vi "Version_4.9_8_on-chip_valves_for25ulSyringe_withModfied_Plunging.vi"() -> ()   [LabVIEW 2020] (continued)
                                n336 = local read "VISA Refnum in\nfor Pump"() -> (w823:refnum<visa-resource-name>)
                                n337 = call "HardStopCurrentProcess (SubVI).vi"("VISA Refnum in"=w823) -> ()  [unwired: 11 in]
                                }
                              }
                              n338 = local read "VISA Refnum in\nfor Pump"() -> (w821:refnum<visa-resource-name>)
                              n339 = call "ProcessCompletionWaiter (SubVI).vi"("VISA Refnum in"=w821) -> ()  [unwired: 11 in]
                            }
                          }
                        }
                      }
                      frame #1 {
                        n340 = local write "Start the Process"(FALSE ("Start the Process")) -> ()
                      }
                    }
                  }
                }
              }
              frame True {
                n341 = local write "Pause Data Collection"(FALSE ("Pause Data Collection")) -> ()
              }
            }
          }
          frame "Initialize Only The Pump" {
            n342 = local read "Stop for End of \nExperiment \nand Data Writing"() -> (w826:bool)
            n343 = case shown="False" w826 {
              frame False {
                n344 = local read "Start the Process"() -> (w827:bool)
                n345 = case shown="True" w827 {
                  frame False {
                    n346 = local read "Stopper that ends \nthe main loops"() -> (w829:bool)
                    n347 = local read "Start the Process"() -> (w830:bool)
                    n348 = Or(x=w830, y=w829) -> (x .or. y?=w828:bool)
                    n349 = case shown="False" w828 {
                      frame False {
                        n350 = while {
                          stop <- w833 stop-if-true
                          n351 = local read "Stopper that ends \nthe main loops"() -> (w835:bool)
                          n352 = local read "Start the Process"() -> (w834:bool)
                          n353 = Or(x=w834, y=w835) -> (x .or. y?=w833:bool)
                          n354 = Wait (ms)(milliseconds to wait=u32 10) -> ()  [unwired: 1 out]
                        }
                        n355 = One Button Dialog(message="Please select the process and press the 'Start Process' Button") -> ()  [unwired: 1 in, 1 out]
                      }
                      frame True {
                      }
                    }
                  }
                  frame True {
                    n356 = stacked-sequence {
                      frame #0 {
                        n357 = local read "VISA Refnum in\nfor Pump"() -> (w836:refnum<visa-resource-name>)
                        n358 = call "Initializer (SubVI).vi"("VISA Refnum in"=w836) -> ()  [unwired: 11 in]
                      }
                      frame #1 {
                        n359 = local read "VISA Refnum in\nfor Pump"() -> (w837:refnum<visa-resource-name>)
                        n360 = call "ProcessCompletionWaiter (SubVI).vi"("VISA Refnum in"=w837) -> ()  [unwired: 11 in]
                      }
                      frame #2 {
                        n361 = local write "Start the Process"(FALSE ("Start the Process")) -> ()
                      }
                    }
                  }
                }
              }
              frame True {
              }
            }
          }
          frame "Automated Protein Purification with 7 SOD Valves and On/Off External Valve" {
            n362 = local read "Stopper that ends \nthe main loops"() -> (w839:bool)
            n363 = case shown="False" w839 {
              frame False {
                n364 = local read "Start the Process"() -> (w840:bool)
                n365 = case shown="True" w840 {
                  frame False {
                    n366 = local read "Stopper that ends \nthe main loops"() -> (w842:bool)
                    n367 = local read "Start the Process"() -> (w841:bool)
                    n368 = Or(x=w842, y=w841) -> (x .or. y?=w843:bool)
                    n369 = case shown="False" w843 {
                      frame False {
                        n370 = while {
                          stop <- w846 stop-if-true
                          n371 = local read "Stop for End of \nExperiment \nand Data Writing"() -> (w845:bool)
                          n372 = local read "Stopper that ends \nthe main loops"() -> (w848:bool)
                          n373 = local read "Start the Process"() -> (w847:bool)
                          n374 = Wait (ms)(milliseconds to wait=u32 10) -> ()  [unwired: 1 out]
                          n375 = Or(x=w848, y=w847) -> (x .or. y?=w846:bool)
                          n376 = local write "Stopper that ends \nthe main loops"(w845) -> ()
                        }
                        n377 = One Button Dialog(message="Please Select the Process and Press 'Start the Process' Button") -> ()  [unwired: 1 in, 1 out]
                      }
                      frame True {
                      }
                    }
                  }
                  frame True {
                    n378 = stacked-sequence {
                      frame #0 {
                        # "Equilibrate Column-1 with Buffer-A obtained from port-4 and pumped via port-2 and Column-2 with Buffer-C obtained from port-4 and pumped onto chip via port-6 onto the chip ...with an initial and inbetween wash of tubings while changing the buffers"
                        n379 = stacked-sequence {
                          frame #0 {
                            n380 = local read "VISA Refnum in\nfor Valve"() -> (w857:refnum<visa-resource-name>)
                            n381 = local read "External Valve \nCLOSED"() -> (w856:string)
                            n382 = local write "Valve V4 Open"(FALSE ("Valve V4 Open")) -> ()
                            n383 = local write "Valve V1 Open"(FALSE ("Valve V1 Open")) -> ()
                            n384 = local write "Valve V2 Open"(FALSE ("Valve V2 Open")) -> ()
                            n385 = local write "Valve V3 Open"(FALSE ("Valve V3 Open")) -> ()
                            n386 = call "PortChanger_Valve (SubVI).vi"("Port Number"=w856, "VISA Refnum in"=w857) -> ()  [unwired: 10 in]
                            n387 = local write "Valve V7 Open"(FALSE ("Valve V7 Open")) -> ()
                            n388 = local write "Valve V5 Open"(FALSE ("Valve V5 Open")) -> ()
                            n389 = local write "Valve V6 Open"(FALSE ("Valve V6 Open")) -> ()
                            n390 = call <vilib>:"fgt init.vi"() -> ("error out"=w852:errorcluster)  [unwired: 11 in]
                            n391 = while {
                              tunnel: w852 -> [w863]
                              tunnel: [w862] -> w851
                              stop <- w866 stop-if-true
                              # "Keeping the valve closing pressure of push pull to zero"
                              n392 = local read "Stop for End of \nExperiment \nand Data Writing"() -> (w867:bool)
                              n393 = local read "Equilibriating \nColumn-1"() -> (w868:bool)
                              n394 = call <vilib>:"fgt set pressure.vi"("error in (no error)"=w863, "pressure"=sgl 0.0 ("order"), "pressureIndex"=1 ("module")) -> ("error out"=w862:errorcluster)  [unwired: 8 in]
                              n395 = Or(x=w868, y=w867) -> (x .or. y?=w866:bool)
                              n396 = Wait (ms)(milliseconds to wait=u32 10) -> ()  [unwired: 1 out]
                            }
                            n397 = call <vilib>:"fgt close.vi"("error in (no error)"=w851) -> ()  [unwired: 10 in, 1 out]
                          }
                          frame #1 {
                            # "Clean the tubing with Buffer-A1"
                            n398 = local read "N-A1"() -> (w870:i32)
                            n399 = for {
                              N: w870 -> [_]
                              n400 = stacked-sequence {
                                frame #0 {
                                n401 = local read "VISA Refnum in\nfor Pump"() -> (w873:refnum<visa-resource-name>)
                                n402 = local read "Port for \nA1-Equilibriation"() -> (w872:string)
                                n403 = call "PortChanger (SubVI).vi"("Port Number"=w872, "VISA Refnum in"=w873) -> ()  [unwired: 10 in]
                                }
                                frame #1 {
                                n404 = local read "VISA Refnum in\nfor Pump"() -> (w874:refnum<visa-resource-name>)
                                n405 = call "ProcessCompletionWaiter (SubVI).vi"("VISA Refnum in"=w874) -> ()  [unwired: 11 in]
                                }
                                frame #2 {
                                n406 = local read "VISA Refnum in\nfor Pump"() -> (w879:refnum<visa-resource-name>)
                                n407 = local read "Apparent Volume\nof Syringe"() -> (w875:dbl)
                                n408 = local read "Volume of Syringe"() -> (w876:dbl)
                                n409 = call "RPickUp(SubVI).vi"("Volume to be picked up"=w875, "Volume of Syringe"=w876, "Resolution of PickUP"=T2."Standard Pumping", "PickUp Flow Rate (ul/min)"=150.0, "VISA Refnum in"=w879) -> ()  [unwired: 6 in, 1 out]
                                }
                                frame #3 {
                                n410 = local read "Stopper that ends \nthe main loops"() -> (w880:bool)
                                n411 = local read "VISA Refnum in\nfor Pump"() -> (w881:refnum<visa-resource-name>)
                                n412 = case shown="True" w880 {
                                frame False {
                                }
                                frame True {
                                n413 = local read "VISA Refnum in\nfor Pump"() -> (w882:refnum<visa-resource-name>)
                                n414 = call "HardStopCurrentProcess (SubVI).vi"("VISA Refnum in"=w882) -> ()  [unwired: 11 in]
                                }
                                }
                                n415 = call "ProcessCompletionWaiter (SubVI).vi"("VISA Refnum in"=w881) -> ()  [unwired: 11 in]
                                }
                                frame #4 {
                                n416 = local read "VISA Refnum in\nfor Pump"() -> (w884:refnum<visa-resource-name>)
                                n417 = call "PortChanger (SubVI).vi"("Port Number"="1", "VISA Refnum in"=w884) -> ()  [unwired: 10 in]
                                }
                                frame #5 {
                                n418 = local read "Stopper that ends \nthe main loops"() -> (w885:bool)
                                n419 = local read "VISA Refnum in\nfor Pump"() -> (w886:refnum<visa-resource-name>)
                                n420 = case shown="True" w885 {
                                frame False {
                                }
                                frame True {
                                n421 = local read "VISA Refnum in\nfor Pump"() -> (w887:refnum<visa-resource-name>)
                                n422 = call "HardStopCurrentProcess (SubVI).vi"("VISA Refnum in"=w887) -> ()  [unwired: 11 in]
                                }
                                }
                                n423 = call "ProcessCompletionWaiter (SubVI).vi"("VISA Refnum in"=w886) -> ()  [unwired: 11 in]
                                }
                                frame #6 {
                                n424 = local read "VISA Refnum in\nfor Pump"() -> (w892:refnum<visa-resource-name>)
                                n425 = local read "Volume of Syringe"() -> (w889:dbl)
                                n426 = call "GoToAbsolutePosition(SubVI).vi"("Absolute Volume Position in Syringe (in ul)"=0.0 ("Volume to be picked up"), "Volume of Syringe"=w889, "Resolution of Pumping"=T2."Standard Pumping" ("Resolution of PickUP"), "Flow Rate (ul/min)"=150.0 ("PickUp Flow Rate (ul/min)"), "VISA Refnum in"=w892) -> ()  [unwired: 6 in, 1 out]
                                }
                                frame #7 {
                                n427 = local read "Stopper that ends \nthe main loops"() -> (w893:bool)
                                n428 = local read "VISA Refnum in\nfor Pump"() -> (w894:refnum<visa-resource-name>)
                                n429 = case shown="True" w893 {
                                frame False {
                                }
                                frame True {
                                n430 = local read "VISA Refnum in\nfor Pump"() -> (w895:refnum<visa-resource-name>)
                                n431 = call "HardStopCurrentProcess (SubVI).vi"("VISA Refnum in"=w895) -> ()  [unwired: 11 in]
                                }
                                }
                                n432 = call "ProcessCompletionWaiter (SubVI).vi"("VISA Refnum in"=w894) -> ()  [unwired: 11 in]
                                }
                              }
                              n433 = local write "Pause Data Collection"(TRUE ("Pause Data Collection")) -> ()
                            }
                          }
                          frame #2 {
                            # "Switch to Port-4"
                            # "Port-4 of pump is connected to Buffer-A1"
                            n434 = local read "Port for \nA1-Equilibriation"() -> (w896:string)
                            n435 = local read "VISA Refnum in\nfor Pump"() -> (w897:refnum<visa-resource-name>)
                            n436 = call "PortChanger (SubVI).vi"("Port Number"=w896, "VISA Refnum in"=w897) -> ()  [unwired: 10 in]
                          }
                          frame #3 {
                            n437 = local read "VISA Refnum in\nfor Pump"() -> (w898:refnum<visa-resource-name>)
                            n438 = call "ProcessCompletionWaiter (SubVI).vi"("VISA Refnum in"=w898) -> ()  [unwired: 11 in]
                          }
                          frame #4 {
                            n439 = local read "VISA Refnum in\nfor Valve"() -> (w905:refnum<visa-resource-name>)
                            n440 = local read "External Valve \nOPEN"() -> (w904:string)
                            n441 = local write "Valve V3 Open"(FALSE ("Valve V3 Open")) -> ()
                            n442 = local write "Valve V4 Open"(FALSE ("Valve V4 Open")) -> ()
                            n443 = local write "Valve V1 Open"(TRUE ("Valve V1 Open")) -> ()
                            n444 = local write "Valve V2 Open"(TRUE ("Valve V2 Open")) -> ()
                            n445 = call "PortChanger_Valve (SubVI).vi"("Port Number"=w904, "VISA Refnum in"=w905) -> ()  [unwired: 10 in]
                            n446 = local write "Valve V6 Open"(FALSE ("Valve V6 Open")) -> ()
                            n447 = local write "Valve V5 Open"(FALSE ("Valve V5 Open")) -> ()
                            n448 = local write "Valve V7 Open"(FALSE ("Valve V7 Open")) -> ()
                          }
                          frame #5 {
                            n449 = local read "Buffer-A1 Volume \nto be  Pumped \nfor Equilibration\nof Column-1"() -> (w911:dbl)
                            n450 = local read "Apparent Volume\nof Syringe"() -> (w908:dbl)
                            n451 = Quotient & Remainder(x=w911, y=w908) -> (x-y*floor(x/y)=w909:dbl, floor(x/y)=w910:dbl)
                            n452 = for {
                              N: w910 -> [_]
                              n453 = stacked-sequence {
                                frame #0 {
                                n454 = local read "Buffer-A1 PickUp \nFlow Rate (ul/min)\nfor Equilibration \nof Column-1"() -> (w914:dbl)
                                n455 = local read "Buffer-A1 Pumping\nResolution \nfor Equilibration \nof Column-1"() -> (w913:T2)
                                n456 = local read "VISA Refnum in\nfor Pump"() -> (w916:refnum<visa-resource-name>)
                                n457 = local read "Apparent Volume\nof Syringe"() -> (w912:dbl)
                                n458 = local read "Volume of Syringe"() -> (w915:dbl)
                                n459 = call "RPickUp(SubVI).vi"("Volume to be picked up"=w912, "Volume of Syringe"=w915, "Resolution of PickUP"=w913, "PickUp Flow Rate (ul/min)"=w914, "VISA Refnum in"=w916) -> ()  [unwired: 6 in, 1 out]
                                }
                                frame #1 {
                                n460 = while {
                                stop <- w917 stop-if-true
                                n461 = local read "Stopper that ends \nthe main loops"() -> (w918:bool)
                                n462 = local read "VISA Refnum in\nfor Pump"() -> (w919:refnum<visa-resource-name>)
                                n463 = case shown="True" w918 {
                                frame False {
                                }
                                frame True {
                                n464 = local read "VISA Refnum in\nfor Pump"() -> (w920:refnum<visa-resource-name>)
                                n465 = call "HardStopCurrentProcess (SubVI).vi"("VISA Refnum in"=w920) -> ()  [unwired: 11 in]
                                }
                                }
                                n466 = call "ProcessCompletionWaiterWithOutPut (SubVI).vi"("VISA Refnum in"=w919) -> ("Boolean"=w917:bool)  [unwired: 10 in]
                                }
                                }
                                frame #2 {
                                # "Reads the initial Plunger Position for computing the volume dispensed"
                                n467 = local read "VISA Refnum in\nfor Pump"() -> (w922:refnum<visa-resource-name>)
                                n468 = call "AbsolutePlungerPosition (SubVI).vi"("VISA Refnum in"=w922) -> ("Plunger Position"=w921:i32)  [unwired: 10 in]
                                n469 = local write "Initial Plunger Position"(w921) -> ()
                                }
                                frame #3 {
                                # "Switch to Port-2"
                                # "Port-2 of the pump is conncted to column-1 of chip"
                                n470 = local read "VISA Refnum in\nfor Pump"() -> (w924:refnum<visa-resource-name>)
                                n471 = call "PortChanger (SubVI).vi"("Port Number"="2", "VISA Refnum in"=w924) -> ()  [unwired: 10 in]
                                }
                                frame #4 {
                                n472 = while {
                                stop <- w925 stop-if-true
                                n473 = local read "Stopper that ends \nthe main loops"() -> (w926:bool)
                                n474 = local read "VISA Refnum in\nfor Pump"() -> (w927:refnum<visa-resource-name>)
                                n475 = case shown="True" w926 {
                                frame False {
                                }
                                frame True {
                                n476 = local read "VISA Refnum in\nfor Pump"() -> (w928:refnum<visa-resource-name>)
                                n477 = call "HardStopCurrentProcess (SubVI).vi"("VISA Refnum in"=w928) -> ()  [unwired: 11 in]
                                }
                                }
                                n478 = call "ProcessCompletionWaiterWithOutPut (SubVI).vi"("VISA Refnum in"=w927) -> ("Boolean"=w925:bool)  [unwired: 10 in]
                                }
                                }
                                frame #5 {
                                n479 = local read "Buffer-A1 Dispense\nFlow Rate (ul/min) \nfor Equilibration\nof Column-1"() -> (w932:dbl)
                                n480 = local read "Buffer-A1 Pumping\nResolution \nfor Equilibration \nof Column-1"() -> (w931:T2)
                                n481 = local read "VISA Refnum in\nfor Pump"() -> (w934:refnum<visa-resource-name>)
                                n482 = local write "Pause Data Collection"(FALSE ("Pause Data Collection")) -> ()
                                n483 = local read "Volume of Syringe"() -> (w933:dbl)
                                n484 = call "GoToAbsolutePosition(SubVI).vi"("Absolute Volume Position in Syringe (in ul)"=0.0, "Volume of Syringe"=w933, "Resolution of Pumping"=w931, "Flow Rate (ul/min)"=w932, "VISA Refnum in"=w934) -> ()  [unwired: 6 in, 1 out]
                                }
                                frame #6 {
                                n485 = local read "Buffer-A1 Pumping\nResolution \nfor Equilibration \nof Column-1"() -> (w936:T2)
                                n486 = local read "VISA Refnum in\nfor Pump"() -> (w938:refnum<visa-resource-name>)
                                n487 = local read "Initial Plunger Position"() -> (w937:dbl)
                                n488 = local read "Volume of Syringe"() -> (w935:dbl)
                                n489 = while {
                                tunnel: w937 -> [w945]
                                tunnel: w938 -> [w944]
                                tunnel: w936 -> [w943]
                                tunnel: w935 -> [w942]
                                stop <- w940 stop-if-true
                                n490 = stacked-sequence {
                                tunnel: w945 -> [w952 _]
                                tunnel: w944 -> [w951 w972]
                                tunnel: w943 -> [w950 _]
                                tunnel: w942 -> [w949 _]
                                tunnel: [_ w970] -> w940
                                frame #0 {
                                n491 = call "AbsolutePlungerPosition (SubVI).vi"("VISA Refnum in"=w951) -> ("Plunger Position"=w948:i32)  [unwired: 10 in]
                                n492 = case shown="\"Standard Pumping\", Default" w950 {
                                tunnel: w952 -> [w957 w966]
                                tunnel: w948 -> [w958 w965]
                                tunnel: [w956 w963] -> w947
                                tunnel: w949 -> [w955 w964]
                                frame "Standard Pumping", Default {
                                n493 = Subtract(x=w957, y=w958) -> (x-y=w954:dbl)
                                n494 = Absolute Value(x=w954) -> (abs(x)=w953:dbl)
                                n495 = Multiply(x=w953, y=w955) -> (x*y=w960:dbl)
                                n496 = Divide(x=w960, y=3000.0) -> (x/y=w956:dbl)
                                }
                                frame "High Resolution Pumping" {
                                n497 = Subtract(x=w966, y=w965) -> (x-y=w962:dbl)
                                n498 = Absolute Value(x=w962) -> (abs(x)=w961:dbl)
                                n499 = Multiply(x=w961, y=w964) -> (x*y=w968:dbl)
                                n500 = Divide(x=w968, y=24000.0) -> (x/y=w963:dbl)
                                }
                                }
                                n501 = local write "Volume being Injected \nin this process"(w947) -> ()
                                }
                                frame #1 {
                                n502 = call "LSPOneStatus (SubVI).vi"("VISA Refnum in"=w972) -> ("read buffer"=w974:string)  [unwired: 10 in]
                                n503 = call <vilib>:"Trim Whitespace.vi"("string"=w974) -> ("trimmed string"=w973:string)  [unwired: 1 in]
                                n504 = local read "Stopper that ends \nthe main loops"() -> (w969:bool)
                                n505 = Equal?(x=w973, y="/0`\u0003") -> (x = y?=w971:bool)
                                n506 = Or(x=w971, y=w969) -> (x .or. y?=w970:bool)
                                }
                                }
                                n507 = Wait (ms)(milliseconds to wait=u32 100) -> ()  [unwired: 1 out]
                                n508 = local read "Stopper that ends \nthe main loops"() -> (w939:bool)
                                n509 = case shown="True" w939 {
                                frame False {
                                }
                                frame True {
                                n510 = local read "VISA Refnum in\nfor Pump"() -> (w946:refnum<visa-resource-name>)
                                n511 = call "HardStopCurrentProcess (SubVI).vi"("VISA Refnum in"=w946) -> ()  [unwired: 11 in]
                                }
                                }
                                }
                                }
                                frame #7 {
                                # "Change the pump port back to Buffer-A1"
                                n512 = local read "VISA Refnum in\nfor Pump"() -> (w977:refnum<visa-resource-name>)
                                n513 = local read "Port for \nA1-Equilibriation"() -> (w976:string)
                                n514 = local write "Pause Data Collection"(TRUE ("Pause Data Collection")) -> ()
                                n515 = Wait (ms)(milliseconds to wait=u32 500) -> ()  [unwired: 1 out]
                                n516 = call "PortChanger (SubVI).vi"("Port Number"=w976, "VISA Refnum in"=w977) -> ()  [unwired: 10 in]
                                }
                                frame #8 {
                                n517 = local read "VISA Refnum in\nfor Pump"() -> (w980:refnum<visa-resource-name>)
                                n518 = local write "Volume being Injected \nin this process"(0.0 ("Volume being Injected \nin this process")) -> ()
                                n519 = call "ProcessCompletionWaiter (SubVI).vi"("VISA Refnum in"=w980) -> ()  [unwired: 11 in]
                                }
                              }
                            }
                            n520 = local write "Reminder of the \nVolume to be \nPumped"(w909) -> ()
                          }
                          frame #6 {
                            n521 = stacked-sequence {
                              frame #0 {
                                n522 = local read "Buffer-A1 PickUp \nFlow Rate (ul/min)\nfor Equilibration \nof Column-1"() -> (w984:dbl)
                                n523 = local read "Buffer-A1 Pumping\nResolution \nfor Equilibration \nof Column-1"() -> (w983:T2)
                                n524 = local read "VISA Refnum in\nfor Pump"() -> (w986:refnum<visa-resource-name>)
                                n525 = local read "Reminder of the \nVolume to be \nPumped"() -> (w982:dbl)
                                n526 = local read "Volume of Syringe"() -> (w985:dbl)
                                n527 = call "RPickUp(SubVI).vi"("Volume to be picked up"=w982, "Volume of Syringe"=w985, "Resolution of PickUP"=w983, "PickUp Flow Rate (ul/min)"=w984, "VISA Refnum in"=w986) -> ()  [unwired: 6 in, 1 out]
                              }
                              frame #1 {
                                n528 = while {
                                stop <- w987 stop-if-true
                                n529 = local read "Stopper that ends \nthe main loops"() -> (w988:bool)
                                n530 = local read "VISA Refnum in\nfor Pump"() -> (w989:refnum<visa-resource-name>)
                                n531 = case shown="True" w988 {
                                frame False {
                                }
                                frame True {
                                n532 = local read "VISA Refnum in\nfor Pump"() -> (w990:refnum<visa-resource-name>)
                                n533 = call "HardStopCurrentProcess (SubVI).vi"("VISA Refnum in"=w990) -> ()  [unwired: 11 in]
                                }
                                }
                                n534 = call "ProcessCompletionWaiterWithOutPut (SubVI).vi"("VISA Refnum in"=w989) -> ("Boolean"=w987:bool)  [unwired: 10 in]
                                }
                              }
                              frame #2 {
                                # "Reads the initial Plunger Position for computing the volume dispensed"
                                n535 = local read "VISA Refnum in\nfor Pump"() -> (w992:refnum<visa-resource-name>)
                                n536 = call "AbsolutePlungerPosition (SubVI).vi"("VISA Refnum in"=w992) -> ("Plunger Position"=w991:i32)  [unwired: 10 in]
                                n537 = local write "Initial Plunger Position"(w991) -> ()
                              }
                              frame #3 {
                                # "Switch to Port-2"
                                # "Port-2 of the pump is conncted to column-1 of chip"
                                n538 = local read "VISA Refnum in\nfor Pump"() -> (w994:refnum<visa-resource-name>)
                                n539 = call "PortChanger (SubVI).vi"("Port Number"="2", "VISA Refnum in"=w994) -> ()  [unwired: 10 in]
                              }
                              frame #4 {
                                n540 = while {
                                stop <- w995 stop-if-true
                                n541 = local read "Stopper that ends \nthe main loops"() -> (w996:bool)
                                n542 = local read "VISA Refnum in\nfor Pump"() -> (w997:refnum<visa-resource-name>)
                                n543 = case shown="True" w996 {
                                frame False {
                                }
                                frame True {
                                n544 = local read "VISA Refnum in\nfor Pump"() -> (w998:refnum<visa-resource-name>)
                                n545 = call "HardStopCurrentProcess (SubVI).vi"("VISA Refnum in"=w998) -> ()  [unwired: 11 in]
                                }
                                }
                                n546 = call "ProcessCompletionWaiterWithOutPut (SubVI).vi"("VISA Refnum in"=w997) -> ("Boolean"=w995:bool)  [unwired: 10 in]
                                }
                              }
                              frame #5 {
                                n547 = local read "Buffer-A1 Pumping\nResolution \nfor Equilibration \nof Column-1"() -> (w1001:T2)
                                n548 = local read "Buffer-A1 Dispense\nFlow Rate (ul/min) \nfor Equilibration\nof Column-1"() -> (w1002:dbl)
                                n549 = local read "VISA Refnum in\nfor Pump"() -> (w1004:refnum<visa-resource-name>)
                                n550 = local write "Pause Data Collection"(FALSE ("Pause Data Collection")) -> ()
                                n551 = local read "Volume of Syringe"() -> (w1003:dbl)
                                n552 = call "GoToAbsolutePosition(SubVI).vi"("Absolute Volume Position in Syringe (in ul)"=0.0 ("Volume to be Dispensed"), "Volume of Syringe"=w1003, "Resolution of Pumping"=w1001, "Flow Rate (ul/min)"=w1002, "VISA Refnum in"=w1004) -> ()  [unwired: 6 in, 1 out]
                              }
                              frame #6 {
                                n553 = local read "Buffer-A1 Pumping\nResolution \nfor Equilibration \nof Column-1"() -> (w1006:T2)
                                n554 = local read "VISA Refnum in\nfor Pump"() -> (w1008:refnum<visa-resource-name>)
                                n555 = local read "Initial Plunger Position"() -> (w1007:dbl)
                                n556 = local read "Volume of Syringe"() -> (w1005:dbl)
                                n557 = while {
                                tunnel: w1007 -> [w1015]
                                tunnel: w1008 -> [w1014]
                                tunnel: w1006 -> [w1013]
                                tunnel: w1005 -> [w1012]
                                stop <- w1010 stop-if-true
                                n558 = stacked-sequence {
                                tunnel: w1015 -> [w1022 _]
                                tunnel: w1014 -> [w1021 w1042]
                                tunnel: w1013 -> [w1020 _]
                                tunnel: w1012 -> [w1019 _]
                                tunnel: [_ w1040] -> w1010
                                frame #0 {
                                n559 = call "AbsolutePlungerPosition (SubVI).vi"("VISA Refnum in"=w1021) -> ("Plunger Position"=w1018:i32)  [unwired: 10 in]
                                n560 = case shown="\"Standard Pumping\", Default" w1020 {
                                tunnel: w1022 -> [w1027 w1036]
                                tunnel: w1018 -> [w1028 w1035]
                                tunnel: [w1026 w1033] -> w1017
                                tunnel: w1019 -> [w1025 w1034]
                                frame "Standard Pumping", Default {
                                n561 = Subtract(x=w1027, y=w1028) -> (x-y=w1024:dbl)
                                n562 = Absolute Value(x=w1024) -> (abs(x)=w1023:dbl)
                                n563 = Multiply(x=w1023, y=w1025) -> (x*y=w1030:dbl)
                                n564 = Divide(x=w1030, y=3000.0) -> (x/y=w1026:dbl)
                                }
                                frame "High Resolution Pumping" {
                                n565 = Subtract(x=w1036, y=w1035) -> (x-y=w1032:dbl)
                                n566 = Absolute Value(x=w1032) -> (abs(x)=w1031:dbl)
                                n567 = Multiply(x=w1031, y=w1034) -> (x*y=w1038:dbl)
                                n568 = Divide(x=w1038, y=24000.0) -> (x/y=w1033:dbl)
                                }
                                }
                                n569 = local write "Volume being Injected \nin this process"(w1017) -> ()
                                }
                                frame #1 {
                                n570 = call "LSPOneStatus (SubVI).vi"("VISA Refnum in"=w1042) -> ("read buffer"=w1044:string)  [unwired: 10 in]
                                n571 = call <vilib>:"Trim Whitespace.vi"("string"=w1044) -> ("trimmed string"=w1043:string)  [unwired: 1 in]
                                n572 = local read "Stopper that ends \nthe main loops"() -> (w1039:bool)
                                n573 = Equal?(x=w1043, y="/0`\u0003") -> (x = y?=w1041:bool)
                                n574 = Or(x=w1041, y=w1039) -> (x .or. y?=w1040:bool)
                                }
                                }
                                n575 = Wait (ms)(milliseconds to wait=u32 100) -> ()  [unwired: 1 out]
                                n576 = local read "Stopper that ends \nthe main loops"() -> (w1009:bool)
                                n577 = case shown="True" w1009 {
                                frame False {
                                }
                                frame True {
                                n578 = local read "VISA Refnum in\nfor Pump"() -> (w1016:refnum<visa-resource-name>)
                                n579 = call "HardStopCurrentProcess (SubVI).vi"("VISA Refnum in"=w1016) -> ()  [unwired: 11 in]
                                }
                                }
                                }
                              }
                              frame #7 {
                                # "Change the pump port to Buffer-C1 for equilibriation of column-2"
                                n580 = local read "VISA Refnum in\nfor Pump"() -> (w1047:refnum<visa-resource-name>)
                                n581 = local read "Port for \nC1-Equilibriation"() -> (w1046:string)
                                n582 = local write "Pause Data Collection"(TRUE ("Pause Data Collection")) -> ()
                                n583 = Wait (ms)(milliseconds to wait=u32 500) -> ()  [unwired: 1 out]
                                n584 = call "PortChanger (SubVI).vi"("Port Number"=w1046, "VISA Refnum in"=w1047) -> ()  [unwired: 10 in]
                              }
                              frame #8 {
                                n585 = local read "VISA Refnum in\nfor Pump"() -> (w1051:refnum<visa-resource-name>)
                                n586 = local write "Volume being Injected \nin this process"(0.0 ("Volume being Injected \nin this process")) -> ()
                                n587 = call "ProcessCompletionWaiter (SubVI).vi"("VISA Refnum in"=w1051) -> ()  [unwired: 11 in]
                                n588 = local write "Start the Process"(FALSE ("Start the Process")) -> ()
                              }
                            }
                          }
                          frame #7 {
                            # "Clean the tubing with Buffer-C1"
                            n589 = local read "N-C1"() -> (w1054:i32)
                            n590 = local write "Equilibriating \nColumn-1"(FALSE ("Equilibriating \nColumn-1")) -> ()
                            n591 = for {
                              N: w1054 -> [_]
                              n592 = stacked-sequence {
                                frame #0 {
                                n593 = local read "Port for \nC1-Equilibriation"() -> (w1057:string)
                                n594 = local read "VISA Refnum in\nfor Pump"() -> (w1058:refnum<visa-resource-name>)
                                n595 = call "PortChanger (SubVI).vi"("Port Number"=w1057, "VISA Refnum in"=w1058) -> ()  [unwired: 10 in]
                                }
                                frame #1 {
                                n596 = local read "VISA Refnum in\nfor Pump"() -> (w1059:refnum<visa-resource-name>)
                                n597 = call "ProcessCompletionWaiter (SubVI).vi"("VISA Refnum in"=w1059) -> ()  [unwired: 11 in]
                                }
                                frame #2 {
                                n598 = local read "VISA Refnum in\nfor Pump"() -> (w1064:refnum<visa-resource-name>)
                                n599 = local read "Apparent Volume\nof Syringe"() -> (w1060:dbl)
                                n600 = local read "Volume of Syringe"() -> (w1061:dbl)
                                n601 = call "RPickUp(SubVI).vi"("Volume to be picked up"=w1060, "Volume of Syringe"=w1061, "Resolution of PickUP"=T2."Standard Pumping", "PickUp Flow Rate (ul/min)"=150.0, "VISA Refnum in"=w1064) -> ()  [unwired: 6 in, 1 out]
                                }
                                frame #3 {
                                n602 = local read "Stopper that ends \nthe main loops"() -> (w1065:bool)
                                n603 = local read "VISA Refnum in\nfor Pump"() -> (w1066:refnum<visa-resource-name>)
                                n604 = case shown="True" w1065 {
                                frame False {
                                }
                                frame True {
                                n605 = local read "VISA Refnum in\nfor Pump"() -> (w1067:refnum<visa-resource-name>)
                                n606 = call "HardStopCurrentProcess (SubVI).vi"("VISA Refnum in"=w1067) -> ()  [unwired: 11 in]
                                }
                                }
                                n607 = call "ProcessCompletionWaiter (SubVI).vi"("VISA Refnum in"=w1066) -> ()  [unwired: 11 in]
                                }
                                frame #4 {
                                n608 = local read "VISA Refnum in\nfor Pump"() -> (w1069:refnum<visa-resource-name>)
                                n609 = call "PortChanger (SubVI).vi"("Port Number"="1", "VISA Refnum in"=w1069) -> ()  [unwired: 10 in]
                                }
                                frame #5 {
                                n610 = local read "Stopper that ends \nthe main loops"() -> (w1070:bool)
                                n611 = local read "VISA Refnum in\nfor Pump"() -> (w1071:refnum<visa-resource-name>)
                                n612 = case shown="True" w1070 {
                                frame False {
                                }
                                frame True {
                                n613 = local read "VISA Refnum in\nfor Pump"() -> (w1072:refnum<visa-resource-name>)
                                n614 = call "HardStopCurrentProcess (SubVI).vi"("VISA Refnum in"=w1072) -> ()  [unwired: 11 in]
                                }
                                }
                                n615 = call "ProcessCompletionWaiter (SubVI).vi"("VISA Refnum in"=w1071) -> ()  [unwired: 11 in]
                                }
                                frame #6 {
                                n616 = local read "VISA Refnum in\nfor Pump"() -> (w1077:refnum<visa-resource-name>)
                                n617 = local read "Volume of Syringe"() -> (w1074:dbl)
                                n618 = call "GoToAbsolutePosition(SubVI).vi"("Absolute Volume Position in Syringe (in ul)"=0.0 ("Volume to be picked up"), "Volume of Syringe"=w1074, "Resolution of Pumping"=T2."Standard Pumping" ("Resolution of PickUP"), "Flow Rate (ul/min)"=150.0 ("PickUp Flow Rate (ul/min)"), "VISA Refnum in"=w1077) -> ()  [unwired: 6 in, 1 out]
                                }
                                frame #7 {
                                n619 = local read "Stopper that ends \nthe main loops"() -> (w1078:bool)
                                n620 = local read "VISA Refnum in\nfor Pump"() -> (w1079:refnum<visa-resource-name>)
                                n621 = case shown="True" w1078 {
                                frame False {
                                }
                                frame True {
                                n622 = local read "VISA Refnum in\nfor Pump"() -> (w1080:refnum<visa-resource-name>)
                                n623 = call "HardStopCurrentProcess (SubVI).vi"("VISA Refnum in"=w1080) -> ()  [unwired: 11 in]
                                }
                                }
                                n624 = call "ProcessCompletionWaiter (SubVI).vi"("VISA Refnum in"=w1079) -> ()  [unwired: 11 in]
                                }
                              }
                            }
                            n625 = local write "Pause Data Collection"(TRUE ("Pause Data Collection")) -> ()
                            n626 = local write "Equilibriating \nColumn-2"(TRUE ("Equilibriating \nColumn-2")) -> ()
                          }
                          frame #8 {
                            n627 = local read "Buffer-C1 Volume \nto be  Pumped \nfor Equilibration\nof Column-2"() -> (w1084:dbl)
                            n628 = local read "Apparent Volume\nof Syringe"() -> (w1081:dbl)
                            n629 = Quotient & Remainder(x=w1084, y=w1081) -> (x-y*floor(x/y)=w1082:dbl, floor(x/y)=w1083:dbl)
                            n630 = for {
                              N: w1083 -> [_]
                              n631 = stacked-sequence {
                                frame #0 {
                                n632 = local read "VISA Refnum in\nfor Pump"() -> (w1086:refnum<visa-resource-name>)
                                n633 = local read "Port for \nC1-Equilibriation"() -> (w1085:string)
                                n634 = call "PortChanger (SubVI).vi"("Port Number"=w1085, "VISA Refnum in"=w1086) -> ()  [unwired: 10 in]
                                }
                                frame #1 {
                                n635 = local read "VISA Refnum in\nfor Pump"() -> (w1087:refnum<visa-resource-name>)
                                n636 = call "ProcessCompletionWaiter (SubVI).vi"("VISA Refnum in"=w1087) -> ()  [unwired: 11 in]
                                }
                                frame #2 {
                                n637 = local read "Buffer-C1 PickUp \nFlow Rate (ul/min)\nfor Equilibration \nof Column-2"() -> (w1090:dbl)
                                n638 = local read "Buffer-C1 Pumping\nResolution \nfor Equilibration \nof Column-2"() -> (w1089:T2)
                                n639 = local read "VISA Refnum in\nfor Pump"() -> (w1092:refnum<visa-resource-name>)
                                n640 = local read "Apparent Volume\nof Syringe"() -> (w1088:dbl)
                                n641 = local read "Volume of Syringe"() -> (w1091:dbl)
                                n642 = call "RPickUp(SubVI).vi"("Volume to be picked up"=w1088, "Volume of Syringe"=w1091, "Resolution of PickUP"=w1089, "PickUp Flow Rate (ul/min)"=w1090, "VISA Refnum in"=w1092) -> ()  [unwired: 6 in, 1 out]
                                }
                                frame #3 {
                                n643 = while {
                                stop <- w1093 stop-if-true
                                n644 = local read "Stopper that ends \nthe main loops"() -> (w1094:bool)
                                n645 = local read "VISA Refnum in\nfor Pump"() -> (w1095:refnum<visa-resource-name>)
                                n646 = case shown="True" w1094 {
                                frame False {
                                }
                                frame True {
                                n647 = local read "VISA Refnum in\nfor Pump"() -> (w1096:refnum<visa-resource-name>)
                                n648 = call "HardStopCurrentProcess (SubVI).vi"("VISA Refnum in"=w1096) -> ()  [unwired: 11 in]
                                }
                                }
                                n649 = call "ProcessCompletionWaiterWithOutPut (SubVI).vi"("VISA Refnum in"=w1095) -> ("Boolean"=w1093:bool)  [unwired: 10 in]
                                }
                                }
                                frame #4 {
                                # "Reads the initial Plunger Position for computing the volume dispensed"
                                n650 = local read "VISA Refnum in\nfor Pump"() -> (w1098:refnum<visa-resource-name>)
                                n651 = call "AbsolutePlungerPosition (SubVI).vi"("VISA Refnum in"=w1098) -> ("Plunger Position"=w1097:i32)  [unwired: 10 in]
                                n652 = local write "Initial Plunger Position"(w1097) -> ()
                                }
                                frame #5 {
                                # "Switch to Port-10"
                                # "Port-10 of the pump is conncted to column-2 of chip"
                                n653 = local read "VISA Refnum in\nfor Pump"() -> (w1100:refnum<visa-resource-name>)
                                n654 = call "PortChanger (SubVI).vi"("Port Number"="10", "VISA Refnum in"=w1100) -> ()  [unwired: 10 in]
                                }
                                frame #6 {
                                n655 = while {
                                stop <- w1101 stop-if-true
                                n656 = local read "Stopper that ends \nthe main loops"() -> (w1102:bool)
                                n657 = local read "VISA Refnum in\nfor Pump"() -> (w1103:refnum<visa-resource-name>)
                                n658 = case shown="True" w1102 {
                                frame False {
                                }
                                frame True {
                                n659 = local read "VISA Refnum in\nfor Pump"() -> (w1104:refnum<visa-resource-name>)
                                n660 = call "HardStopCurrentProcess (SubVI).vi"("VISA Refnum in"=w1104) -> ()  [unwired: 11 in]
                                }
                                }
                                n661 = call "ProcessCompletionWaiterWithOutPut (SubVI).vi"("VISA Refnum in"=w1103) -> ("Boolean"=w1101:bool)  [unwired: 10 in]
                                }
                                }
                                frame #7 {
                                # "Buffer-C pumped for column non-interference"
                                # "Keeps the AMF valve after column-1 open and valve after column-2 closed"
                                n662 = local read "Buffer-C1 Dispense\nFlow Rate (ul/min) \nfor Equilibration\nof Column-2"() -> (w1117:dbl)
                                n663 = local read "Buffer-C1 Pumping\nResolution \nfor Equilibration \nof Column-2"() -> (w1116:T2)
                                n664 = local read "VISA Refnum in\nfor Pump"() -> (w1119:refnum<visa-resource-name>)
                                n665 = local write "Pause Data Collection"(FALSE ("Pause Data Collection")) -> ()
                                n666 = local read "Volume of Syringe"() -> (w1118:dbl)
                                n667 = call "GoToAbsolutePosition(SubVI).vi"("Absolute Volume Position in Syringe (in ul)"=0.0, "Volume of Syringe"=w1118, "Resolution of Pumping"=w1116, "Flow Rate (ul/min)"=w1117, "VISA Refnum in"=w1119) -> ()  [unwired: 6 in, 1 out]
                                n668 = local write "Valve V1 Open"(FALSE ("Valve V1 Open")) -> ()
                                n669 = local write "Valve V2 Open"(TRUE ("Valve V2 Open")) -> ()
                                n670 = local write "Valve V4 Open"(FALSE ("Valve V4 Open")) -> ()
                                n671 = local write "Valve V3 Open"(TRUE ("Valve V3 Open")) -> ()
                                n672 = local read "VISA Refnum in\nfor Valve"() -> (w1110:refnum<visa-resource-name>)
                                n673 = local read "External Valve \nOPEN"() -> (w1109:string)
                                n674 = local write "Valve V5 Open"(FALSE ("Valve V5 Open")) -> ()
                                n675 = local write "Valve V6 Open"(FALSE ("Valve V6 Open")) -> ()
                                n676 = local write "Valve V7 Open"(FALSE ("Valve V7 Open")) -> ()
                                n677 = call "PortChanger_Valve (SubVI).vi"("Port Number"=w1109, "VISA Refnum in"=w1110) -> ()  [unwired: 10 in]
                                }
                                frame #8 {
                                n678 = local read "Buffer-C1 Pumping\nResolution \nfor Equilibration \nof Column-2"() -> (w1121:T2)
                                n679 = local read "VISA Refnum in\nfor Pump"() -> (w1123:refnum<visa-resource-name>)
                                n680 = local read "Initial Plunger Position"() -> (w1122:dbl)
                                n681 = local read "Volume of Syringe"() -> (w1120:dbl)
                                n682 = while {
                                tunnel: w1122 -> [w1130]
                                tunnel: w1123 -> [w1129]
                                tunnel: w1121 -> [w1128]
                                tunnel: w1120 -> [w1127]
                                stop <- w1125 stop-if-true
                                n683 = stacked-sequence {
                                tunnel: w1130 -> [w1137 _]
                                tunnel: w1129 -> [w1136 w1161]
                                tunnel: w1128 -> [w1135 _]
                                tunnel: w1127 -> [w1134 _]
                                tunnel: [_ w1159] -> w1125
                                frame #0 {
                                n684 = call "AbsolutePlungerPosition (SubVI).vi"("VISA Refnum in"=w1136) -> ("Plunger Position"=w1133:i32)  [unwired: 10 in]
                                n685 = case shown="\"Standard Pumping\", Default" w1135 {
                                tunnel: w1137 -> [w1142 w1151]
                                tunnel: w1133 -> [w1143 w1150]
                                tunnel: [w1141 w1148] -> w1132
                                tunnel: w1134 -> [w1140 w1149]
                                frame "Standard Pumping", Default {
                                n686 = Subtract(x=w1142, y=w1143) -> (x-y=w1139:dbl)
                                n687 = Absolute Value(x=w1139) -> (abs(x)=w1138:dbl)
                                n688 = Multiply(x=w1138, y=w1140) -> (x*y=w1145:dbl)
                                n689 = Divide(x=w1145, y=3000.0) -> (x/y=w1141:dbl)
                                }
                                frame "High Resolution Pumping" {
                                n690 = Subtract(x=w1151, y=w1150) -> (x-y=w1147:dbl)
                                n691 = Absolute Value(x=w1147) -> (abs(x)=w1146:dbl)
                                n692 = Multiply(x=w1146, y=w1149) -> (x*y=w1153:dbl)
                                n693 = Divide(x=w1153, y=24000.0) -> (x/y=w1148:dbl)
                                }
                                }
                                n694 = local write "Volume being Injected \nin this process"(w1132) -> ()
                                }
                                frame #1 {
                                n695 = local read "Buffer-C Volume \nto be Pumped for\nColumn \nnon-interference"() -> (w1157:dbl)
                                n696 = local read "Volume being Injected \nin this process"() -> (w1158:dbl)
                                n697 = local read "Stopper that ends \nthe main loops"() -> (w1156:bool)
                                n698 = call "LSPOneStatus (SubVI).vi"("VISA Refnum in"=w1161) -> ("read buffer"=w1163:string)  [unwired: 10 in]
                                n699 = call <vilib>:"Trim Whitespace.vi"("string"=w1163) -> ("trimmed string"=w1162:string)  [unwired: 1 in]
                                n700 = Equal?(x=w1162, y="/0`\u0003") -> (x = y?=w1160:bool)
                                n701 = Greater Or Equal?(x=w1158, y=w1157) -> (x >= y?=w1155:bool)
                                n702 = Or(x=w1156, y=w1155) -> (x .or. y?=w1154:bool)
                                n703 = Or(x=w1160, y=w1154) -> (x .or. y?=w1159:bool)
                                }
                                }
                                n704 = Wait (ms)(milliseconds to wait=u32 100) -> ()  [unwired: 1 out]
                                n705 = local read "Stopper that ends \nthe main loops"() -> (w1124:bool)
                                n706 = case shown="True" w1124 {
                                frame False {
                                }
                                frame True {
                                n707 = local read "VISA Refnum in\nfor Pump"() -> (w1131:refnum<visa-resource-name>)
                                n708 = call "HardStopCurrentProcess (SubVI).vi"("VISA Refnum in"=w1131) -> ()  [unwired: 11 in]
                                }
                                }
                                }
                                }
                                frame #9 {
                                # "Keeps the AMF valve after column-1 closed and valve after column-2 open"
                                n709 = local read "VISA Refnum in\nfor Valve"() -> (w1169:refnum<visa-resource-name>)
                                n710 = local read "External Valve \nCLOSED"() -> (w1168:string)
                                n711 = local write "Valve V3 Open"(FALSE ("Valve V3 Open")) -> ()
                                n712 = local write "Valve V2 Open"(FALSE ("Valve V2 Open")) -> ()
                                n713 = local write "Valve V4 Open"(TRUE ("Valve V1 Open")) -> ()
                                n714 = local write "Valve V1 Open"(FALSE ("Valve V1 Open")) -> ()
                                n715 = call "PortChanger_Valve (SubVI).vi"("Port Number"=w1168, "VISA Refnum in"=w1169) -> ()  [unwired: 10 in]
                                n716 = local write "Valve V5 Open"(TRUE ("Valve V4 Open")) -> ()
                                n717 = local write "Valve V7 Open"(TRUE ("Valve V6 Open")) -> ()
                                n718 = local write "Valve V6 Open"(FALSE ("Valve V6 Open")) -> ()
                                }
                                frame #10 {
                                n719 = local read "Buffer-C1 Pumping\nResolution \nfor Equilibration \nof Column-2"() -> (w1175:T2)
                                n720 = local read "VISA Refnum in\nfor Pump"() -> (w1177:refnum<visa-resource-name>)
                                n721 = local read "Initial Plunger Position"() -> (w1176:dbl)
                                n722 = local read "Volume of Syringe"() -> (w1174:dbl)
                                n723 = while {
                                tunnel: w1176 -> [w1184]
                                tunnel: w1177 -> [w1183]
                                tunnel: w1175 -> [w1182]
                                tunnel: w1174 -> [w1181]
                                stop <- w1179 stop-if-true
                                n724 = stacked-sequence {
                                tunnel: w1184 -> [w1191 _]
                                tunnel: w1183 -> [w1190 w1211]
                                tunnel: w1182 -> [w1189 _]
                                tunnel: w1181 -> [w1188 _]
                                tunnel: [_ w1209] -> w1179
                                frame #0 {
                                n725 = call "AbsolutePlungerPosition (SubVI).vi"("VISA Refnum in"=w1190) -> ("Plunger Position"=w1187:i32)  [unwired: 10 in]
                                n726 = case shown="\"Standard Pumping\", Default" w1189 {
                                tunnel: w1191 -> [w1196 w1205]
                                tunnel: w1187 -> [w1197 w1204]
                                tunnel: [w1195 w1202] -> w1186
                                tunnel: w1188 -> [w1194 w1203]
                                frame "Standard Pumping", Default {
                                n727 = Subtract(x=w1196, y=w1197) -> (x-y=w1193:dbl)
                                n728 = Absolute Value(x=w1193) -> (abs(x)=w1192:dbl)
                                n729 = Multiply(x=w1192, y=w1194) -> (x*y=w1199:dbl)
                                n730 = Divide(x=w1199, y=3000.0) -> (x/y=w1195:dbl)
                                }
                                frame "High Resolution Pumping" {
                                n731 = Subtract(x=w1205, y=w1204) -> (x-y=w1201:dbl)
                                n732 = Absolute Value(x=w1201) -> (abs(x)=w1200:dbl)
                                n733 = Multiply(x=w1200, y=w1203) -> (x*y=w1207:dbl)
                                n734 = Divide(x=w1207, y=24000.0) -> (x/y=w1202:dbl)
                                }
                                }
                                n735 = local write "Volume being Injected \nin this process"(w1186) -> ()
                                }
                                frame #1 {
                                n736 = local read "Stopper that ends \nthe main loops"() -> (w1208:bool)
                                n737 = call "LSPOneStatus (SubVI).vi"("VISA Refnum in"=w1211) -> ("read buffer"=w1213:string)  [unwired: 10 in]
                                n738 = call <vilib>:"Trim Whitespace.vi"("string"=w1213) -> ("trimmed string"=w1212:string)  [unwired: 1 in]
                                n739 = Equal?(x=w1212, y="/0`\u0003") -> (x = y?=w1210:bool)
                                n740 = Or(x=w1210, y=w1208) -> (x .or. y?=w1209:bool)
                                }
                                }
                                n741 = Wait (ms)(milliseconds to wait=u32 100) -> ()  [unwired: 1 out]
                                n742 = local read "Stopper that ends \nthe main loops"() -> (w1178:bool)
                                n743 = case shown="True" w1178 {
                                frame False {
                                }
                                frame True {
                                n744 = local read "VISA Refnum in\nfor Pump"() -> (w1185:refnum<visa-resource-name>)
                                n745 = call "HardStopCurrentProcess (SubVI).vi"("VISA Refnum in"=w1185) -> ()  [unwired: 11 in]
                                }
                                }
                                }
                                }
                                frame #11 {
                                # "Change the pump port back to Buffer-C1"
                                n746 = local read "VISA Refnum in\nfor Pump"() -> (w1216:refnum<visa-resource-name>)
                                n747 = local read "Port for \nC1-Equilibriation"() -> (w1215:string)
                                n748 = local write "Pause Data Collection"(TRUE ("Pause Data Collection")) -> ()
                                n749 = Wait (ms)(milliseconds to wait=u32 500) -> ()  [unwired: 1 out]
                                n750 = call "PortChanger (SubVI).vi"("Port Number"=w1215, "VISA Refnum in"=w1216) -> ()  [unwired: 10 in]
                                }
                                frame #12 {
                                n751 = local read "VISA Refnum in\nfor Pump"() -> (w1219:refnum<visa-resource-name>)
                                n752 = local write "Volume being Injected \nin this process"(0.0 ("Volume being Injected \nin this process")) -> ()
                                n753 = call "ProcessCompletionWaiter (SubVI).vi"("VISA Refnum in"=w1219) -> ()  [unwired: 11 in]
                                }
                              }
                            }
                            n754 = local write "Reminder of the \nVolume to be \nPumped"(w1082) -> ()
                          }
                          frame #9 {
                            n755 = stacked-sequence {
                              frame #0 {
                                n756 = local read "Buffer-C1 PickUp \nFlow Rate (ul/min)\nfor Equilibration \nof Column-2"() -> (w1223:dbl)
                                n757 = local read "Buffer-C1 Pumping\nResolution \nfor Equilibration \nof Column-2"() -> (w1222:T2)
                                n758 = local read "VISA Refnum in\nfor Pump"() -> (w1225:refnum<visa-resource-name>)
                                n759 = local read "Reminder of the \nVolume to be \nPumped"() -> (w1221:dbl)
                                n760 = local read "Volume of Syringe"() -> (w1224:dbl)
                                n761 = call "RPickUp(SubVI).vi"("Volume to be picked up"=w1221, "Volume of Syringe"=w1224, "Resolution of PickUP"=w1222, "PickUp Flow Rate (ul/min)"=w1223, "VISA Refnum in"=w1225) -> ()  [unwired: 6 in, 1 out]
                              }
                              frame #1 {
                                n762 = while {
                                stop <- w1226 stop-if-true
                                n763 = local read "Stopper that ends \nthe main loops"() -> (w1227:bool)
                                n764 = local read "VISA Refnum in\nfor Pump"() -> (w1228:refnum<visa-resource-name>)
                                n765 = case shown="True" w1227 {
                                frame False {
                                }
                                frame True {
                                n766 = local read "VISA Refnum in\nfor Pump"() -> (w1229:refnum<visa-resource-name>)
                                n767 = call "HardStopCurrentProcess (SubVI).vi"("VISA Refnum in"=w1229) -> ()  [unwired: 11 in]
                                }
                                }
                                n768 = call "ProcessCompletionWaiterWithOutPut (SubVI).vi"("VISA Refnum in"=w1228) -> ("Boolean"=w1226:bool)  [unwired: 10 in]
                                }
                              }
                              frame #2 {
                                # "Reads the initial Plunger Position for computing the volume dispensed"
                                n769 = local read "VISA Refnum in\nfor Pump"() -> (w1231:refnum<visa-resource-name>)
                                n770 = call "AbsolutePlungerPosition (SubVI).vi"("VISA Refnum in"=w1231) -> ("Plunger Position"=w1230:i32)  [unwired: 10 in]
                                n771 = local write "Initial Plunger Position"(w1230) -> ()
                              }
                              frame #3 {
                                # "Switch to Port-10"
                                # "Port-10 of the pump is conncted to column-2 of chip"
                                n772 = local read "VISA Refnum in\nfor Pump"() -> (w1233:refnum<visa-resource-name>)
                                n773 = call "PortChanger (SubVI).vi"("Port Number"="10", "VISA Refnum in"=w1233) -> ()  [unwired: 10 in]
                              }
                              frame #4 {
                                n774 = while {
                                stop <- w1234 stop-if-true
                                n775 = local read "Stopper that ends \nthe main loops"() -> (w1235:bool)
                                n776 = local read "VISA Refnum in\nfor Pump"() -> (w1236:refnum<visa-resource-name>)
                                n777 = case shown="True" w1235 {
                                frame False {
                                }
                                frame True {
                                n778 = local read "VISA Refnum in\nfor Pump"() -> (w1237:refnum<visa-resource-name>)
                                n779 = call "HardStopCurrentProcess (SubVI).vi"("VISA Refnum in"=w1237) -> ()  [unwired: 11 in]
                                }
                                }
                                n780 = call "ProcessCompletionWaiterWithOutPut (SubVI).vi"("VISA Refnum in"=w1236) -> ("Boolean"=w1234:bool)  [unwired: 10 in]
                                }
                              }
                              frame #5 {
                                # "Keeps the AMF valve after column-1 open and valve after column-2 closed"
                                n781 = local read "Buffer-C1 Dispense\nFlow Rate (ul/min) \nfor Equilibration\nof Column-2"() -> (w1250:dbl)
                                n782 = local read "Buffer-C1 Pumping\nResolution \nfor Equilibration \nof Column-2"() -> (w1249:T2)
                                n783 = local read "VISA Refnum in\nfor Pump"() -> (w1252:refnum<visa-resource-name>)
                                n784 = local write "Pause Data Collection"(FALSE ("Pause Data Collection")) -> ()
                                n785 = local read "Volume of Syringe"() -> (w1251:dbl)
                                n786 = call "GoToAbsolutePosition(SubVI).vi"("Absolute Volume Position in Syringe (in ul)"=0.0, "Volume of Syringe"=w1251, "Resolution of Pumping"=w1249, "Flow Rate (ul/min)"=w1250, "VISA Refnum in"=w1252) -> ()  [unwired: 6 in, 1 out]
                                n787 = local read "VISA Refnum in\nfor Valve"() -> (w1242:refnum<visa-resource-name>)
                                n788 = local write "Valve V1 Open"(FALSE ("Valve V1 Open")) -> ()
                                n789 = local write "Valve V2 Open"(TRUE ("Valve V2 Open")) -> ()
                                n790 = local write "Valve V3 Open"(TRUE ("Valve V3 Open")) -> ()
                                n791 = local write "Valve V4 Open"(FALSE ("Affinity On")) -> ()
                                n792 = local read "External Valve \nOPEN"() -> (w1241:string)
                                n793 = local write "Valve V5 Open"(FALSE ("Valve V5 Open")) -> ()
                                n794 = local write "Valve V6 Open"(FALSE ("Valve V6 Open")) -> ()
                                n795 = local write "Valve V7 Open"(FALSE ("Valve V7 Open")) -> ()
                                n796 = call "PortChanger_Valve (SubVI).vi"("Port Number"=w1241, "VISA Refnum in"=w1242) -> ()  [unwired: 10 in]
                              }
                              frame #6 {
                                n797 = local read "Buffer-C1 Pumping\nResolution \nfor Equilibration \nof Column-2"() -> (w1254:T2)
                                n798 = local read "VISA Refnum in\nfor Pump"() -> (w1256:refnum<visa-resource-name>)
                                n799 = local read "Initial Plunger Position"() -> (w1255:dbl)
                                n800 = local read "Volume of Syringe"() -> (w1253:dbl)
                                n801 = while {
                                tunnel: w1255 -> [w1263]
                                tunnel: w1256 -> [w1262]
                                tunnel: w1254 -> [w1261]
                                tunnel: w1253 -> [w1260]
                                stop <- w1258 stop-if-true
                                n802 = stacked-sequence {
                                tunnel: w1263 -> [w1270 _]
                                tunnel: w1262 -> [w1269 w1294]
                                tunnel: w1261 -> [w1268 _]
                                tunnel: w1260 -> [w1267 _]
                                tunnel: [_ w1292] -> w1258
                                frame #0 {
                                n803 = call "AbsolutePlungerPosition (SubVI).vi"("VISA Refnum in"=w1269) -> ("Plunger Position"=w1266:i32)  [unwired: 10 in]
                                n804 = case shown="\"Standard Pumping\", Default" w1268 {
                                tunnel: w1270 -> [w1275 w1284]
                                tunnel: w1266 -> [w1276 w1283]
                                tunnel: [w1274 w1281] -> w1265
                                tunnel: w1267 -> [w1273 w1282]
                                frame "Standard Pumping", Default {
                                n805 = Subtract(x=w1275, y=w1276) -> (x-y=w1272:dbl)
                                n806 = Absolute Value(x=w1272) -> (abs(x)=w1271:dbl)
                                n807 = Multiply(x=w1271, y=w1273) -> (x*y=w1278:dbl)
                                n808 = Divide(x=w1278, y=3000.0) -> (x/y=w1274:dbl)
